vi "Read Pin Map.vi"(8 "error in (no error)":errorcluster, 11 "NI-DAQ in":refnum<class "NI-DAQ.lvclass">) -> (0 "error out":errorcluster, 2 "Pin Map":T1={"Region Valves"=[49, 52, 0, 0], "Extra Valves"=[[[0.0, 48.0, 0.0, 0.0, 0.0]]], "Tool Primary Valve"=51, "Tool Secondary Valve"=50, "Region Sensors"=[37, 41, 37], "Extra Sensors"=[[[36.0, 37.0, 0.0, 0.0]]], "Tool Primary Sensor"=39.0, "Tool Secondary Sensor"=38.0, "Compression Sensor"=31.0, "5V"=50}, 3 "NI-DAQ out":refnum<class "NI-DAQ.lvclass">)   [LabVIEW 2019, in "NI-DAQ.lvclass"]
uses:
  NI-DAQ.lvclass
  Pin Map.ctl
  I-O.lvclass
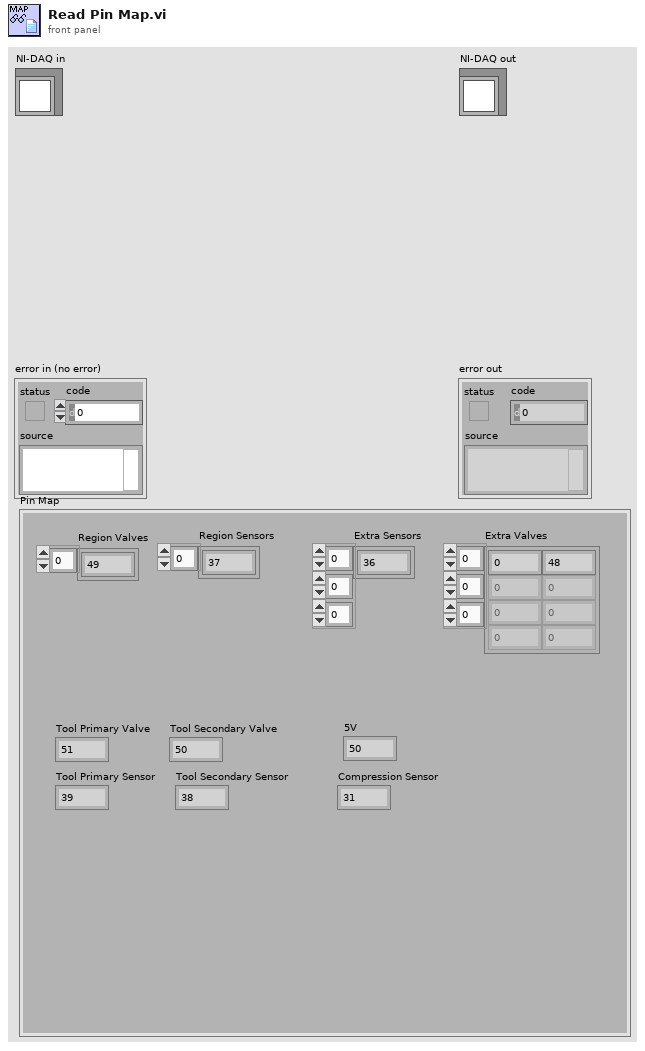
[diagram p1: front panel]
types:
  T1 = typedef "I-O.lvclass/Pin Map.ctl" = cluster{"Region Valves":i32[], "Extra Valves":dbl[][][], "Tool Primary Valve":i32, "Tool Secondary Valve":i32, "Region Sensors":i32[], "Extra Sensors":dbl[][][], "Tool Primary Sensor":dbl, "Tool Secondary Sensor":dbl, "Compression Sensor":dbl, "5V":i32}
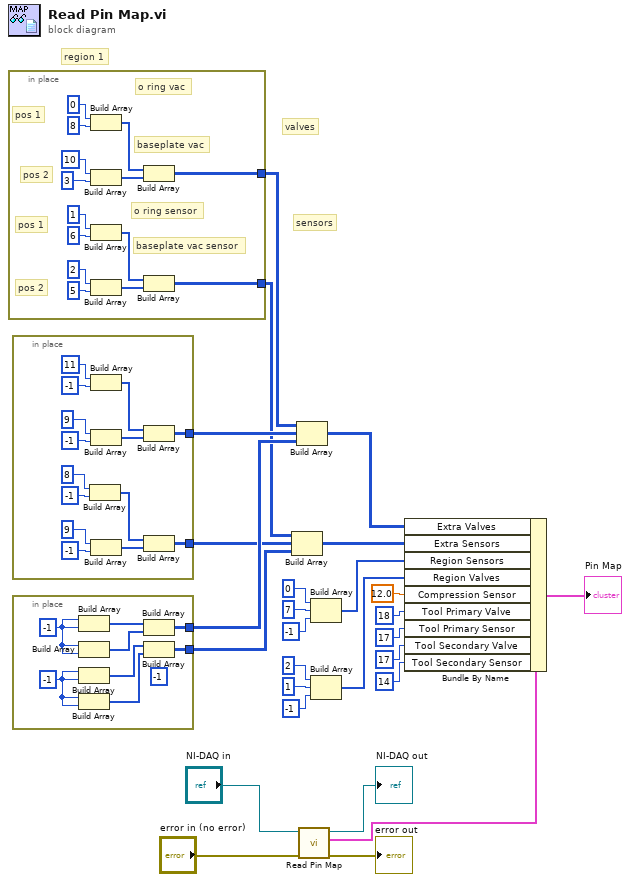
[diagram p0: block diagram]
diagram:
  # "sensors"
  # "valves"
  # "region 1"
  n1 = in-place {
    in-place-border: [w35] -> w8
    in-place-border: [w28] -> w5
    # "pos 2"
    # "baseplate vac sensor"
    # "o ring sensor"
    # "pos 1"
    # "pos 2"
    # "baseplate vac"
    # "o ring vac"
    # "pos 1"
    n2 = Build Array(0, 8) -> (w36:i32[])
    n3 = Build Array(10, 3) -> (w37:i32[])
    n4 = Build Array(1, 6) -> (w29:i32[])
    n5 = Build Array(2, 5) -> (w30:i32[])
    n6 = Build Array(w36, w37) -> (w35:i32[][])
    n7 = Build Array(w29, w30) -> (w28:i32[][])
  }
  n8 = in-place {
    in-place-border: [w49] -> w7
    in-place-border: [w42] -> w4
    n9 = Build Array(8, -1) -> (w44:i32[])
    n10 = Build Array(11, -1) -> (w51:i32[])
    n11 = Build Array(9, -1) -> (w50:i32[])
    n12 = Build Array(9, -1) -> (w43:i32[])
    n13 = Build Array(w51, w50) -> (w49:i32[][])
    n14 = Build Array(w44, w43) -> (w42:i32[][])
  }
  n15 = in-place {
    in-place-border: [w60] -> w6
    in-place-border: [w57] -> w3
    w56 = -1
    (unwired) -1
    w62 = -1
    n16 = Build Array(w62, w62) -> (w63:i32[])
    n17 = Build Array(w62, w62) -> (w61:i32[])
    n18 = Build Array(w56, w56) -> (w59:i32[])
    n19 = Build Array(w56, w56) -> (w58:i32[])
    n20 = Build Array(w63, w61) -> (w60:i32[][])
    n21 = Build Array(w59, w58) -> (w57:i32[][])
  }
  n22 = Build Array(w5, w4, w3) -> (w1:i32[][][])
  n23 = Build Array(w8, w7, w6) -> (w2:i32[][][])
  n24 = call-parent "Read Pin Map.vi"("error in (no error)"="error in (no error)", "I-O in"="NI-DAQ in") -> ("error out"=→"error out":errorcluster, "Pin Map 2"=w23:T1, "I-O out"=→"NI-DAQ out":refnum<class "NI-DAQ.lvclass">)  [unwired: 7 in]
  n25 = Build Array(0, 7, -1) -> (w9:i32[])
  n26 = Build Array(2, 1, -1) -> (w15:i32[])
  n27 = Bundle By Name(cluster=w23, "Extra Valves"=w2, "Extra Sensors"=w1, "Region Sensors"=w9, "Region Valves"=w15, "Compression Sensor"=12.0, "Tool Primary Valve"=18, "Tool Primary Sensor"=17 ("Tool Primary Valve"), "Tool Secondary Valve"=17 ("Tool Primary Valve"), "Tool Secondary Sensor"=14 ("Tool Secondary Valve")) -> (→"Pin Map":T1)
